vi "To Variant.vi"(0 "Obj in":refnum<class "FSM.Edge.lvclass">, 11 "error in (no error)":errorcluster) -> (4 "Obj out":refnum<class "FSM.Edge.lvclass">, 8 "Array":variant[](array[variant]), 15 "error out":errorcluster)   [LabVIEW 2020, in "FSM.Edge.lvclass"]
uses:
  FSM.Edge.lvclass
  FSM.Edge.lvclass/FSM.Edge.ctl
  epl-vi-lib/Koop/KObject Class/KObject.lvclass
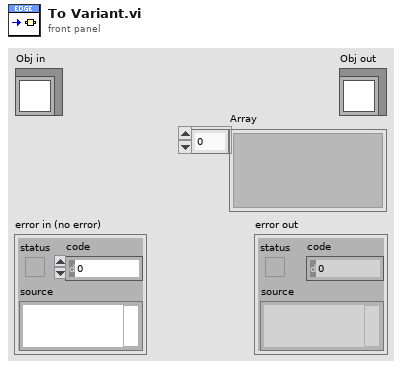
[diagram p1: front panel]
types:
  T1 = typedef "FSM.Edge.lvclass/Serialized.ctl" = cluster{"Label":refnum<class "FSM.Label.lvclass">, "SourceName":string, "TargetName":string, "Points":cluster{"x":i16, "y":i16}[], "Color":u32, "Style":enum32{"Solid", "Dash", "Dot", "DashDot", "DashDotDot"}, "SourceEnd":refnum<class "FSM.EdgeEnd.lvclass">, "TargetEnd":refnum<class "FSM.EdgeEnd.lvclass">, "Type":string, "Annotations":refnum<class "FSM.Annotation.lvclass">}
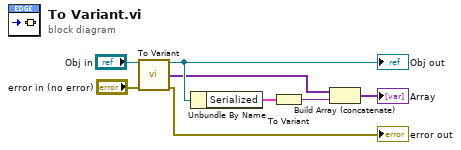
[diagram p0: block diagram]
diagram:
  n1 = call-parent "To Variant.vi"("KObject in"="Obj in", "error in (no error)"="error in (no error)") -> ("KObject out"=w3:refnum<class "FSM.Edge.lvclass">, "Array"=w2:variant[], "error out"=→"error out":errorcluster)  [unwired: 11 in]
  "Obj out" <- w3
  n2 = Unbundle By Name(w3) -> ("Serialized"=w4:T1)
  n3 = To Variant(anything=w4) -> (Variant=w5:variant)
  n4 = Build Array (concatenate)(w2, w5) -> (→"Array":variant[])
